vi "Test Voltage Command.vi"(11 "Test Case In":refnum<class "Test Commands.lvclass">) -> (0 "error out":errorcluster, 3 "Test Case Out":refnum<class "Test Commands.lvclass">)   [LabVIEW 2019, in "Test Commands.lvclass"]
uses:
  Test Commands.lvclass
  C:/Program Files (x86)/National Instruments/LabVIEW 2024/vi.lib/Astemes/LUnit/Test Case.lvclass
  <vilib>/Astemes/LUnit/Test Case.lvclass/Test Case.ctl
  4993e8ee-a06a-463a-9684-69129f64d5ce.vi
  <vilib>/Astemes/LUnit/Core/LUnit Test Case/Private/Append Pass Result.vi
  <vilib>/Astemes/LUnit/Core/LUnit Test Case/Private/Append Fail Result.vi
  4993e8ee-a06a-463a-9684-69129f64d5ce.vi/9c5d11cd-9439-4240-a1ee-d9baace9c924.vi
  <vilib>/Astemes/LUnit/Core/LUnit Test Case/Private/Run In UI.vi
  <vilib>/Utility/error.llb/Clear Errors.vi
  Libraries/Inversor/Inversor.lvlib
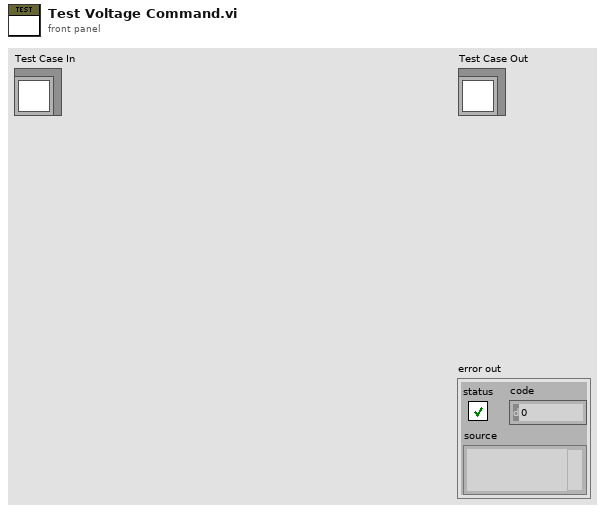
[diagram p1: front panel]
types:
  T1 = enum16{"Set Voltage", "Set Frecuency", "Set Speed", "Set Current"}
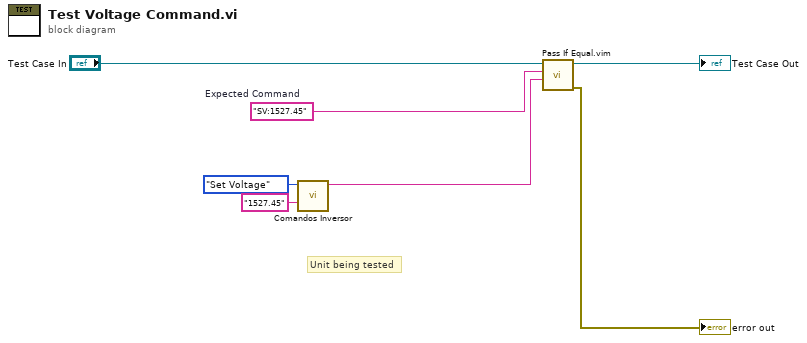
[diagram p0: block diagram]
diagram:
  w1 = "SV:1527.45"  # Expected Command
  # "Unit being tested"
  n1 = call "Comandos Inversor.vi"("Argument"="1527.45", "Command"=T1."Set Voltage") -> ("Command"=w2:string)  [unwired: 9 in]
  n2 = call "Pass If Equal.vim"("Actual"=w2, "Expected"=w1, "LUnit Test Case In"="Test Case In") -> ("error out"=→"error out":errorcluster, "LUnit Test Case Out"=→"Test Case Out":refnum<class "Test Commands.lvclass">)  [unwired: 7 in]
